vi "Read_userEventInstances.vi"(8 "error in (no error)":errorcluster, 11 "tcpServer in":refnum<class "TcpServer.lvclass">) -> (0 "error out":errorcluster, 2 "UserEvents":T1, 3 "tcpServer out":refnum<class "TcpServer.lvclass">)   [LabVIEW 2018, in "TcpServer.lvclass"]
doc: "Read UserEvent cluster, with user event instances inside."
uses:
  TcpServer.lvclass
  typedef/userEventsTypeDef.ctl
  typedef/ackTypeDef.ctl
  TcpServer.lvclass/TcpServer.ctl
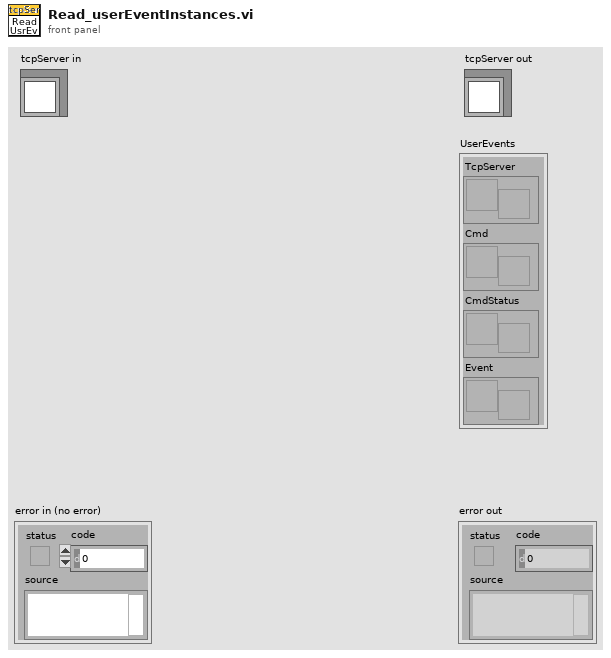
[diagram p1: front panel]
types:
  T1 = typedef "TcpServer.lvclass/userEventsTypeDef.ctl" = cluster{"TcpServer":refnum<user-event>, "Cmd":refnum<user-event>, "CmdStatus":refnum<user-event>, "Event":refnum<user-event>}
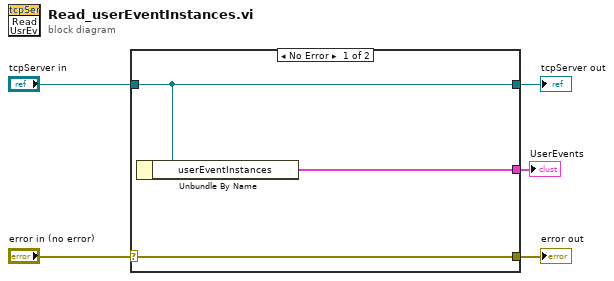
[diagram p0: block diagram]
diagram:
  n1 = case shown="No Error" "error in (no error)" {
    selector: "error in (no error)" -> [w8 w9]
    tunnel: [w8 w9] -> w4
    tunnel: [w7 w10] -> w2
    tunnel: "tcpServer in" -> [w7 w10]
    tunnel: [w6 _] -> w1
    frame No Error {
      n2 = Unbundle By Name(w7) -> ("userEventInstances"=w6:T1)
    }
    frame Error {
    }
  }
  "error out" <- w4
  "tcpServer out" <- w2
  "UserEvents" <- w1
